vi "set execution system.vi"(10 "execution system":T1, 11 "task in":refnum<class "task.lvclass">) -> (3 "task out":refnum<class "task.lvclass">)   [LabVIEW 2013, in "task.lvclass"]
uses:
  task.lvclass
  dispatcher/execution system.ctl
  task.lvclass/task.ctl
  dispatcher/thread pool.lvclass
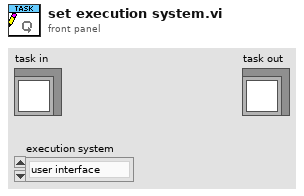
[diagram p1: front panel]
types:
  T1 = typedef "thread pool.lvclass/execution system.ctl" = enum32{"user interface", "standard", "instrument i/o", "data acquisition", "other 1", "other 2"}
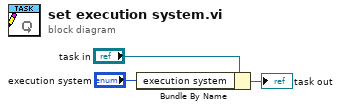
[diagram p0: block diagram]
diagram:
  n1 = Bundle By Name(cluster="task in", "execution system"="execution system") -> (→"task out":refnum<class "task.lvclass">)
